vi "Write_tcpListenerID.vi"(8 "error in (no error)":errorcluster, 10 "tcpListenerID":refnum<k5>, 11 "TcpServerBase in":refnum<class "TcpServerBase.lvclass">) -> (0 "error out":errorcluster, 3 "TcpServerBase out":refnum<class "TcpServerBase.lvclass">)   [LabVIEW 2018, in "TcpServerBase.lvclass"]
doc: "Write the TCP Listener ID after the TCP Create Listener function is executed."
uses:
  TcpServerBase.lvclass
  TcpServerBase.lvclass/TcpServerBase.ctl
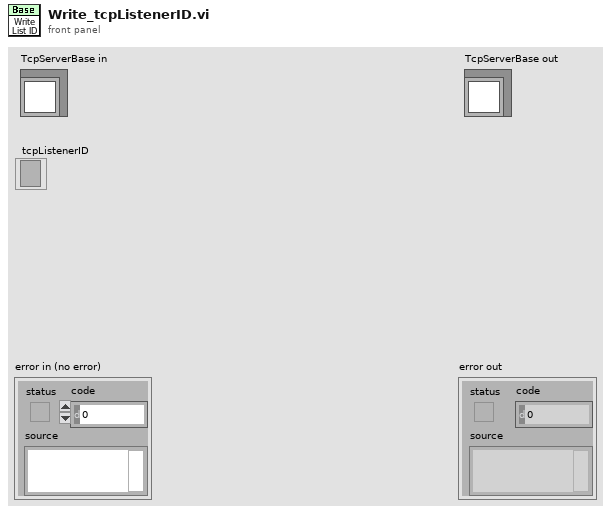
[diagram p1: front panel]
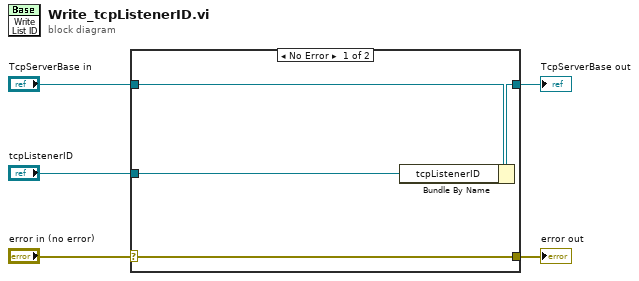
[diagram p0: block diagram]
diagram:
  n1 = case shown="No Error" "error in (no error)" {
    selector: "error in (no error)" -> [w9 w10]
    tunnel: [w9 w10] -> w4
    tunnel: [w7 w11] -> w2
    tunnel: "TcpServerBase in" -> [w8 w11]
    tunnel: "tcpListenerID" -> [w6 _]
    frame No Error {
      n2 = Bundle By Name(cluster=w8, "tcpListenerID"=w6) -> (w7:refnum<class "TcpServerBase.lvclass">)
    }
    frame Error {
    }
  }
  "error out" <- w4
  "TcpServerBase out" <- w2
